vi "Main_Simulator_10Pixels.vi"() -> ()   [LabVIEW 2015]
doc: "Demonstrates the fundamentals of the State Machine design pattern in LabVIEW. A state machine, in its simplest form, is a case structure within a while loop, with a state enum wired to a shift register on the loop to define the execution of different cases (or \"states\") of the case structure on different iterations of the loop."
uses:
  State Machine Fundamentals - State Enum.ctl
panel:
  in  "Play Back Speed":u32(slide) scale=0.0..10.0
  out "subarray 10":string[](array[string])
  out "subarray 9":string[](array[string])
  out "subarray 8":string[](array[string])
  out "subarray 7":string[](array[string])
  out "subarray 6":string[](array[string])
  out "subarray 5":string[](array[string])
  out "subarray 4":string[](array[string])
  out "subarray 3":string[](array[string])
  out "subarray 2":string[](array[string])
  out "subarray":string[](array[string])
  out "INDEX":i32
  in  "ALL":u32(colorbox)=16448250
  in  "SET ALL":bool
  in  "LED STRIP 1":T1={"Pixel 0"=16448250, "Pixel 1"=16448250, "Pixel 2"=16448250, "Pixel 3"=16448250, "Pixel 4"=16448250, "Pixel 5"=16448250, "Pixel 6"=16448250, "Pixel 7"=16448250, "Pixel 8"=16448250, "Pixel 9"=16448250}
  in  "Stop":bool
  in  "RUN":bool
  in  "SET":bool
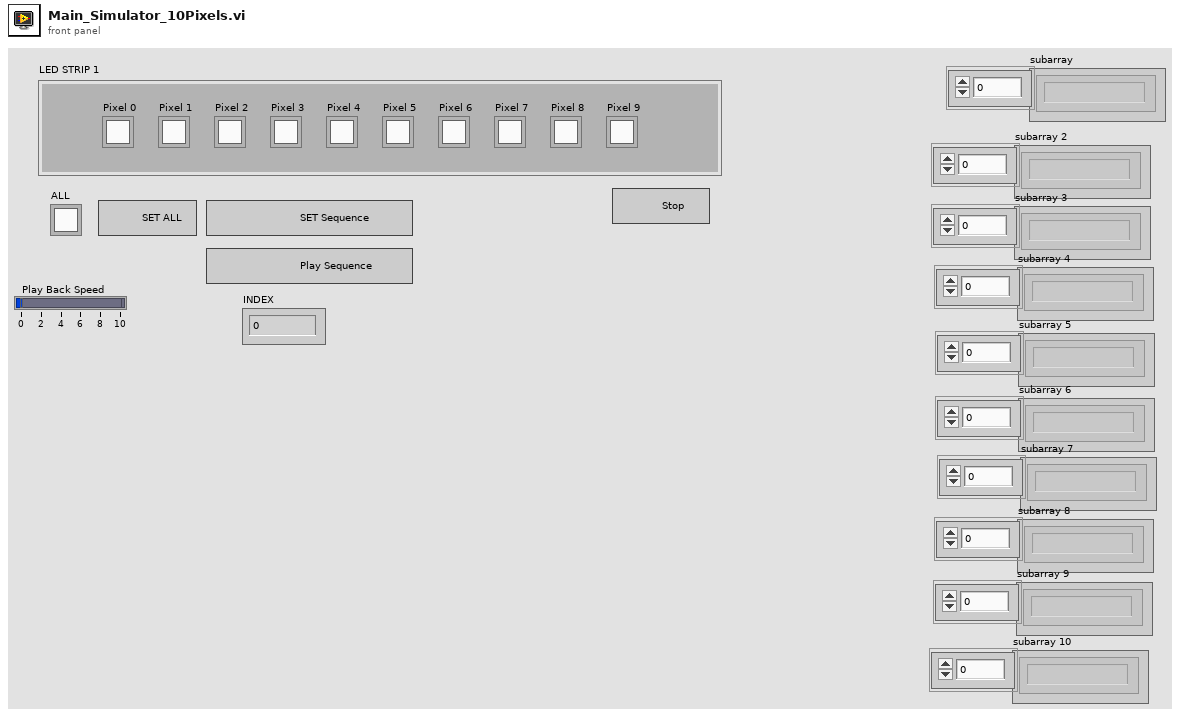
[diagram p1: front panel]
types:
  T1 = cluster{"Pixel 0":u32, "Pixel 1":u32, "Pixel 2":u32, "Pixel 3":u32, "Pixel 4":u32, "Pixel 5":u32, "Pixel 6":u32, "Pixel 7":u32, "Pixel 8":u32, "Pixel 9":u32}
  T2 = cluster{"Pixel 9":u32, "Pixel 8":u32, "Pixel 7":u32, "Pixel 6":u32, "Pixel 5":u32, "Pixel 4":u32, "Pixel 3":u32, "Pixel 2":u32, "Pixel 1":u32, "Pixel 0":u32}
  T3 = typedef "State Machine Fundamentals - State Enum.ctl" = enum16{"Initialize", "Wait for Event", "SET", "PLAY", "Stop"}
  T4 = cluster{"String Array OUT":string[][], "Index":i32, "Current Array":u32[], "LED STRIP 2":cluster{"Pixel 9":u32, "Pixel 8":u32, "Pixel 7":u32, "Pixel 6":u32, "Pixel 5":u32, "Pixel 4":u32, "Pixel 3":u32, "Pixel 2":u32, "Pixel 1":u32, "Pixel 0":u32}}
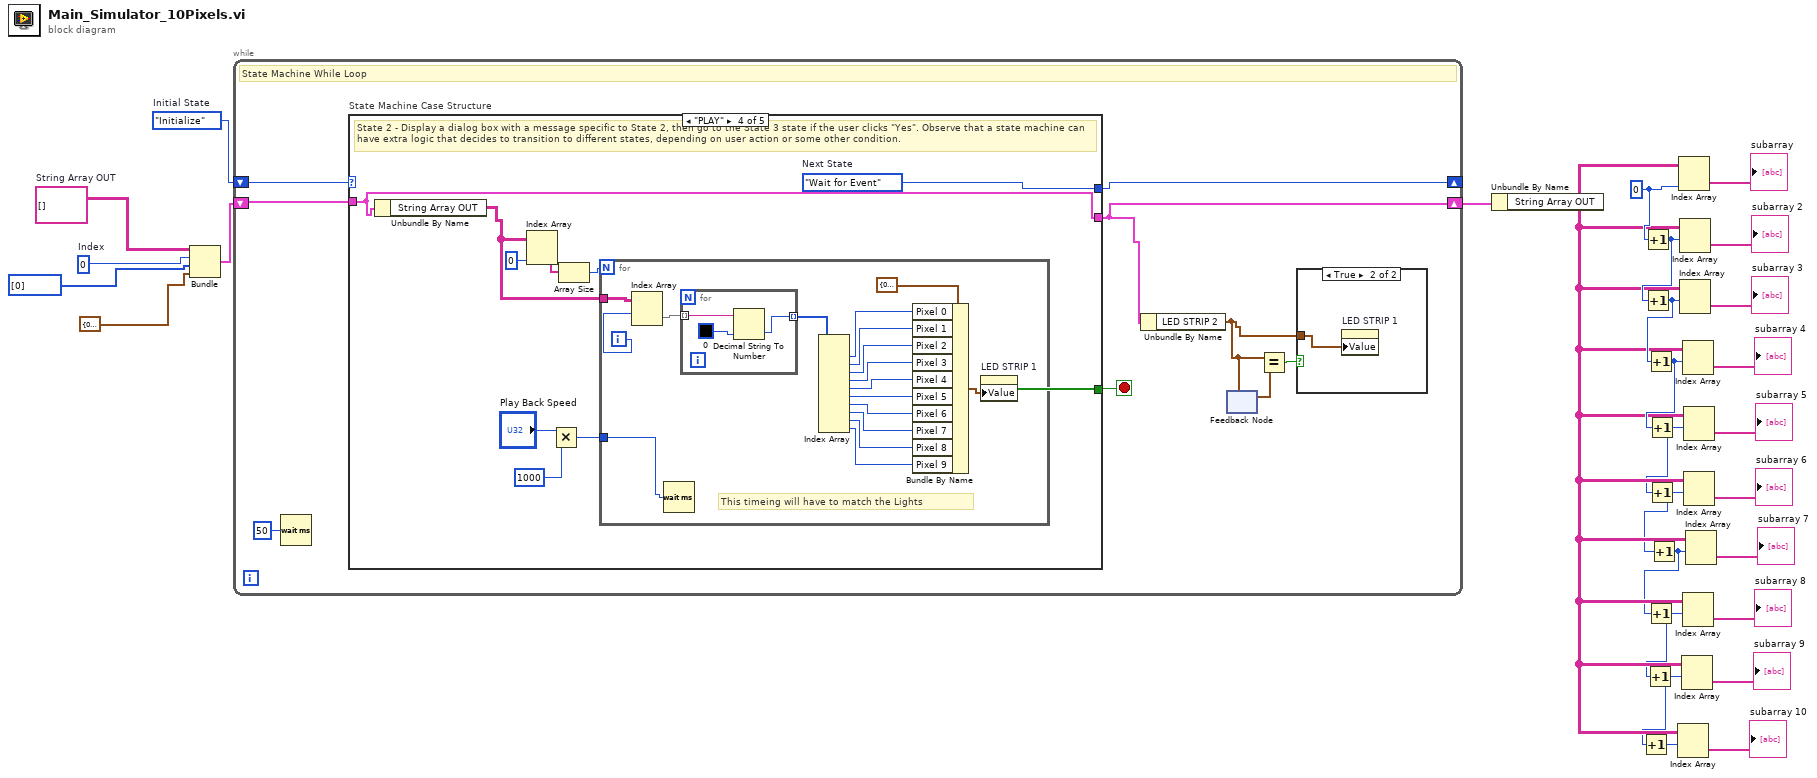
[diagram p0: block diagram]
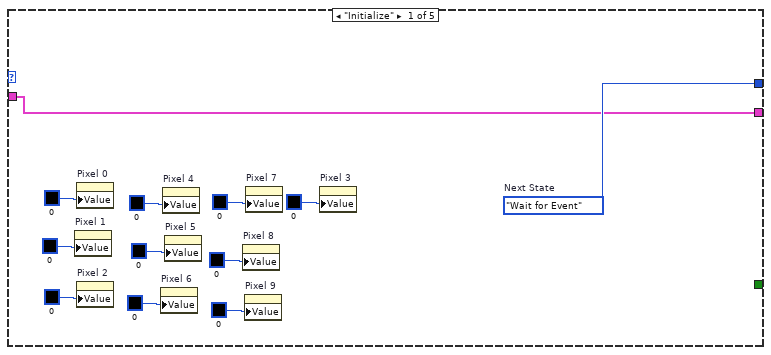
[diagram p3: hidden frame]
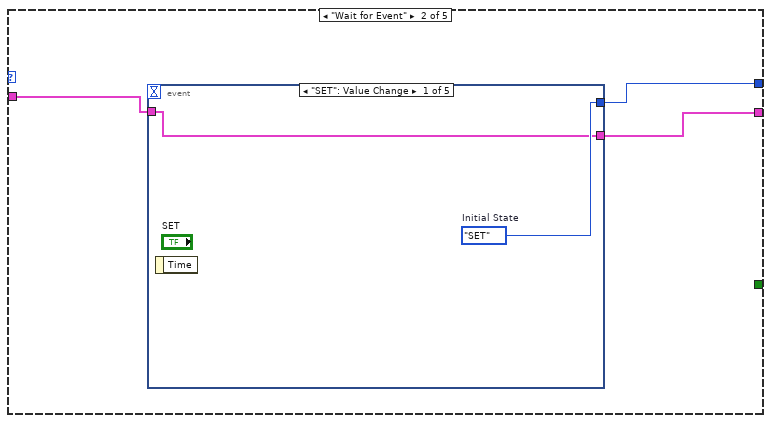
[diagram p4: hidden frame]
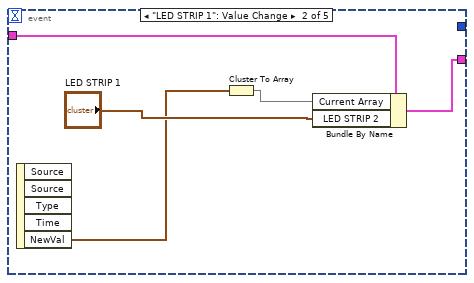
[diagram p5: hidden frame]
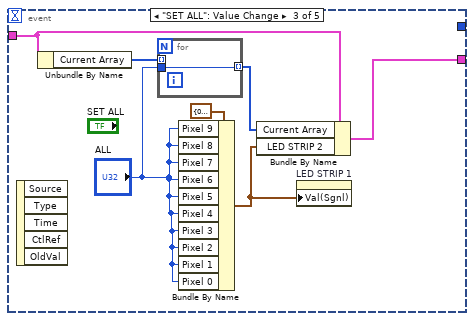
[diagram p6: hidden frame]
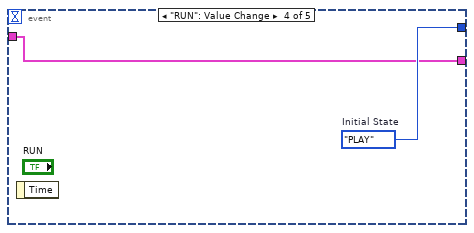
[diagram p7: hidden frame]
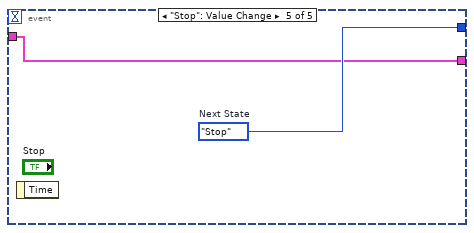
[diagram p8: hidden frame]
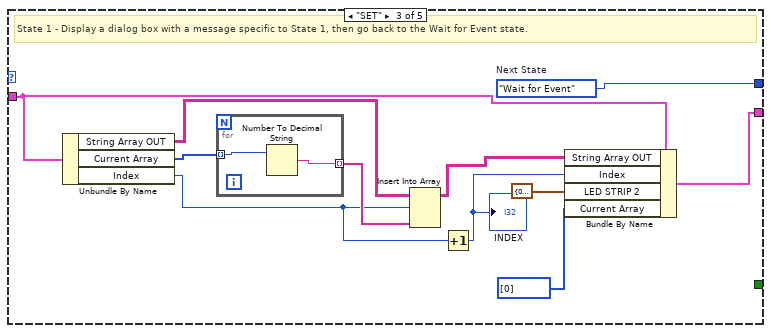
[diagram p9: hidden frame]
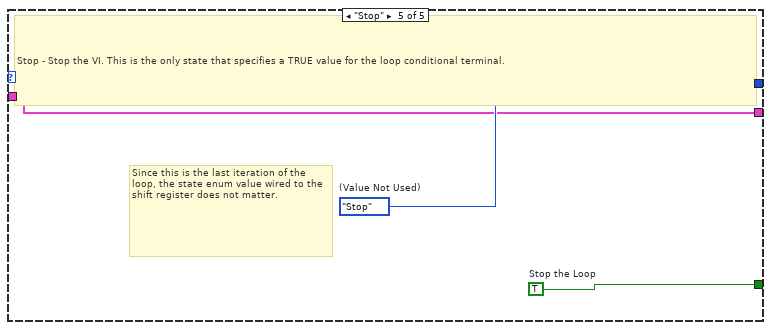
[diagram p10: hidden frame]
diagram:
  w19 = 0 ("disabled index (col)")
  w25 = 0  # Index
  w26 = string[][] []  # String Array OUT
  w28 = State_Machine_Fundamentals_-_State_Enum."Initialize"  # Initial State
  n1 = Bundle("String Array OUT"=w26, "Index"=w25, "Current Array"=u32[] [0], "LED STRIP 2"=T2 {"Pixel 9"=0, "Pixel 8"=0, "Pixel 7"=0, "Pixel 6"=0, "Pixel 5"=0, "Pixel 4"=0, "Pixel 3"=0, "Pixel 2"=0, "Pixel 1"=0, "Pixel 0"=0}) -> (w27:T4)  [unwired: 1 in]
  n2 = while {
    shift-right: [w36] -> _
    shift-left: w28 -> [w37]
    shift-right: [w33] -> w22
    shift-left: w27 -> [w34]
    stop <- w35 stop-if-true
    # "State Machine While Loop"
    n3 = Wait (ms)(milliseconds to wait=u32 50) -> ()  [unwired: 1 out]
    n4 = case "State Machine Case Structure" shown="\"PLAY\"" w37 {
      tunnel: [w50 w53 w83 w92 w117] -> w36
      tunnel: [_ _ _ _ w116] -> w35
      tunnel: w34 -> [w49 w52 w79 w93 w115]
      tunnel: [w49 w51 w78 w93 w115] -> w33
      frame "Initialize" {
        w50 = State_Machine_Fundamentals_-_State_Enum."Wait for Event"  # Next State
        n5 = property on="Pixel 1" class="ColBox"("Value"=u32 0 ("Pixel 0")) -> ()  [unwired: 2 in, 2 out]
        n6 = property on="Pixel 0" class="ColBox"("Value"=u32 0 ("Pixel 0")) -> ()  [unwired: 2 in, 2 out]
        n7 = property on="Pixel 2" class="ColBox"("Value"=u32 0 ("Pixel 0")) -> ()  [unwired: 2 in, 2 out]
        n8 = property on="Pixel 6" class="ColBox"("Value"=u32 0 ("Pixel 0")) -> ()  [unwired: 2 in, 2 out]
        n9 = property on="Pixel 4" class="ColBox"("Value"=u32 0 ("Pixel 0")) -> ()  [unwired: 2 in, 2 out]
        n10 = property on="Pixel 5" class="ColBox"("Value"=u32 0 ("Pixel 0")) -> ()  [unwired: 2 in, 2 out]
        n11 = property on="Pixel 8" class="ColBox"("Value"=u32 0 ("Pixel 0")) -> ()  [unwired: 2 in, 2 out]
        n12 = property on="Pixel 9" class="ColBox"("Value"=u32 0 ("Pixel 0")) -> ()  [unwired: 2 in, 2 out]
        n13 = property on="Pixel 7" class="ColBox"("Value"=u32 0 ("Pixel 0")) -> ()  [unwired: 2 in, 2 out]
        n14 = property on="Pixel 3" class="ColBox"("Value"=u32 0 ("Pixel 0")) -> ()  [unwired: 2 in, 2 out]
      }
      frame "Wait for Event" {
        n15 = event shown="[0] \"SET\": Value Change" {
          selector: _ -> [_ _ _ _ _]
          dyn-events: _ -> [_ _ _ _ _]
          timeout: _ -> [_ _ _ _ _]
          tunnel: [w55 _ _ w70 w72] -> w53
          tunnel: w52 -> [w54 w60 w65 w69 w71]
          tunnel: [w54 w59 w67 w69 w71] -> w51
          event "SET": Value Change {
            w55 = State_Machine_Fundamentals_-_State_Enum."SET"  # Initial State
            n16 = event-data() -> ()  [unwired: 1 in, 1 out]
          }
          event "LED STRIP 1": Value Change {
            n17 = event-data() -> ("NewVal"=w56:T1)  [unwired: 1 in, 4 out]
            n18 = Cluster To Array(cluster=w56) -> (array=w57:u32[])
            n19 = Bundle By Name(cluster=w60, "Current Array"=w57, "LED STRIP 2"="LED STRIP 1") -> (w59:T4)
          }
          event "SET ALL": Value Change {
            n20 = event-data() -> ()  [unwired: 1 in, 5 out]
            n21 = Unbundle By Name(w65) -> ("Current Array"=w64:u32[])
            n22 = for {
              tunnel: "ALL" -> [w68]
              tunnel: w64 -> [_] mode=indexing
              tunnel: [w68] -> w63 mode=indexing
            }
            n23 = Bundle By Name(cluster=T2 {"Pixel 9"=0, "Pixel 8"=0, "Pixel 7"=0, "Pixel 6"=0, "Pixel 5"=0, "Pixel 4"=0, "Pixel 3"=0, "Pixel 2"=0, "Pixel 1"=0, "Pixel 0"=0} ("LED STRIP 2"), "Pixel 9"="ALL", "Pixel 8"="ALL", "Pixel 7"="ALL", "Pixel 6"="ALL", "Pixel 5"="ALL", "Pixel 4"="ALL", "Pixel 3"="ALL", "Pixel 2"="ALL", "Pixel 1"="ALL", "Pixel 0"="ALL") -> (w61:T2)
            n24 = Bundle By Name(cluster=w65, "Current Array"=w63, "LED STRIP 2"=w61) -> (w67:T4)
            n25 = property on="LED STRIP 1" class="Clust (strict)"("Val(Sgnl)"=w61) -> ()  [unwired: 2 in, 2 out]
          }
          event "RUN": Value Change {
            w70 = State_Machine_Fundamentals_-_State_Enum."PLAY"  # Initial State
            n26 = event-data() -> ()  [unwired: 1 in, 1 out]
          }
          event "Stop": Value Change {
            w72 = State_Machine_Fundamentals_-_State_Enum."Stop"  # Next State
            n27 = event-data() -> ()  [unwired: 1 in, 1 out]
          }
        }
      }
      frame "SET" {
        w83 = State_Machine_Fundamentals_-_State_Enum."Wait for Event"  # Next State
        # "State 1 - Display a dialog box with a message specific to State 1, then go back to the Wait for Event state."
        n28 = Unbundle By Name(w79) -> ("String Array OUT"=w80:string[][], "Current Array"=w81:u32[], "Index"=w73:i32)
        n29 = for {
          tunnel: w81 -> [w85] mode=indexing
          tunnel: [w84] -> w82 mode=indexing
          n30 = Number To Decimal String(number=w85) -> (decimal integer string=w84:string)  [unwired: 1 in]
        }
        n31 = Insert Into Array(array=w80, index (row)=w73, new element=w82) -> (w77:string[][])  [unwired: 1 in]
        n32 = Increment(x=w73) -> (x+1=w76:i32)
        "INDEX" <- w76
        n33 = Bundle By Name(cluster=w79, "String Array OUT"=w77, "Index"=w76, "LED STRIP 2"=T2 {"Pixel 9"=0, "Pixel 8"=0, "Pixel 7"=0, "Pixel 6"=0, "Pixel 5"=0, "Pixel 4"=0, "Pixel 3"=0, "Pixel 2"=0, "Pixel 1"=0, "Pixel 0"=0}, "Current Array"=u32[] [0]) -> (w78:T4)
      }
      frame "PLAY" {
        w92 = State_Machine_Fundamentals_-_State_Enum."Wait for Event"  # Next State
        # "State 2 - Display a dialog box with a message specific to State 2, then go to the State 3 state if the user clicks \"Yes\". Observe that a state machine can have extra logic that decides to transition to different states, depending on user action or some other condition."
        n34 = Unbundle By Name(w93) -> ("String Array OUT"=w94:string[][])
        n35 = Index Array(array=w94, index (col)=0 ("disabled index (col)")) -> (element=w90:string[])  [unwired: 1 in]
        n36 = Multiply(x="Play Back Speed", y=u32 1000) -> (x*y=w86:u32)
        n37 = Array Size(array=w90) -> (size(s)=w89:i32)
        n38 = for {
          N: w89 -> [_]
          tunnel: w94 -> [w110]
          tunnel: w86 -> [w95]
          i -> [w97]
          # "This timeing will have to match the Lights"
          n39 = Index Array(array=w110, index (row)=w97) -> (element=w109:string[])  [unwired: 1 in]
          n40 = Wait (ms)(milliseconds to wait=w95) -> ()  [unwired: 1 out]
          n41 = for {
            tunnel: w109 -> [w114] mode=indexing
            tunnel: [w112] -> w111 mode=indexing
            n42 = Decimal String To Number(string=w114, default (0L)=u32 0 ("Pixel 5")) -> (number=w112:u32)  [unwired: 1 in, 1 out]
          }
          n43 = Index Array(array=w111) -> (element #1=w107:u32, element #2=w106:u32, element #3=w105:u32, element #4=w104:u32, element #5=w103:u32, element #6=w102:u32, element #7=w101:u32, element #8=w100:u32, element #9=w99:u32, element #10=w98:u32)  [unwired: 10 in]
          n44 = Bundle By Name(cluster=T1 {"Pixel 0"=0, "Pixel 1"=0, "Pixel 2"=0, "Pixel 3"=0, "Pixel 4"=0, "Pixel 5"=0, "Pixel 6"=0, "Pixel 7"=0, "Pixel 8"=0, "Pixel 9"=0} ("LED STRIP 1"), "Pixel 0"=w107, "Pixel 1"=w106, "Pixel 2"=w105, "Pixel 3"=w104, "Pixel 4"=w103, "Pixel 5"=w102, "Pixel 6"=w101, "Pixel 7"=w100, "Pixel 8"=w99, "Pixel 9"=w98) -> (w96:T1)
          n45 = property on="LED STRIP 1" class="Clust (strict)"("Value"=w96) -> ()  [unwired: 2 in, 2 out]
        }
      }
      frame "Stop" {
        w116 = TRUE  # Stop the Loop
        w117 = State_Machine_Fundamentals_-_State_Enum."Stop"  # (Value Not Used)
        # "Since this is the last iteration of the loop, the state enum value wired to the shift register does not matter."
        # "Stop - Stop the VI. This is the only state that specifies a TRUE value for the loop conditional terminal."
      }
    }
    n46 = Unbundle By Name(w33) -> ("LED STRIP 2"=w29:T2)
    n47 = feedback-in #1(w29) -> ()
    n48 = feedback #1() -> (w32:T2)  [unwired: 1 in]
    n49 = Equal?(x=w29, y=w32) -> (x = y?=w31:bool)
    n50 = case shown="True" w31 {
      tunnel: w29 -> [_ w38]
      frame False {
      }
      frame True {
        n51 = property on="LED STRIP 1" class="Clust (strict)"("Value"=w38) -> ()  [unwired: 2 in, 2 out]
      }
    }
  }
  n52 = Unbundle By Name(w22) -> ("String Array OUT"=w6:string[][])
  n53 = Increment(x=w19) -> (x+1=w9:i32)
  n54 = Increment(x=w9) -> (x+1=w8:i32)
  n55 = Increment(x=w8) -> (x+1=w7:i32)
  n56 = Increment(x=w7) -> (x+1=w5:i32)
  n57 = Increment(x=w5) -> (x+1=w4:i32)
  n58 = Increment(x=w4) -> (x+1=w3:i32)
  n59 = Increment(x=w3) -> (x+1=w2:i32)
  n60 = Increment(x=w2) -> (x+1=w1:i32)
  n61 = Increment(x=w1) -> (x+1=w10:i32)
  n62 = Index Array(array=w6, index (row)=w10) -> (element=→"subarray 10":string[])  [unwired: 1 in]
  n63 = Index Array(array=w6, index (col)=w19) -> (element=→"subarray":string[])  [unwired: 1 in]
  n64 = Index Array(array=w6, index (row)=w9) -> (element=→"subarray 2":string[])  [unwired: 1 in]
  n65 = Index Array(array=w6, index (row)=w8) -> (element=→"subarray 3":string[])  [unwired: 1 in]
  n66 = Index Array(array=w6, index (row)=w1) -> (element=→"subarray 9":string[])  [unwired: 1 in]
  n67 = Index Array(array=w6, index (row)=w7) -> (element=→"subarray 4":string[])  [unwired: 1 in]
  n68 = Index Array(array=w6, index (row)=w2) -> (element=→"subarray 8":string[])  [unwired: 1 in]
  n69 = Index Array(array=w6, index (row)=w5) -> (element=→"subarray 5":string[])  [unwired: 1 in]
  n70 = Index Array(array=w6, index (row)=w4) -> (element=→"subarray 6":string[])  [unwired: 1 in]
  n71 = Index Array(array=w6, index (row)=w3) -> (element=→"subarray 7":string[])  [unwired: 1 in]
